vi "final.vi"() -> ()   [LabVIEW 2019]
uses:
  <vilib>/userdefined/High Color/IMAQdx.ctl
  <vilib>/DAQmx/write.llb/DAQmx Write (Digital 1D Bool NChan 1Samp 1Line).vi
  <vilib>/DAQmx/read.llb/DAQmx Read (Digital 1D Bool NChan 1Samp 1Line).vi
  <vilib>/Instr/_visa.llb/VISA Configure Serial Port (Instr).vi
  <vilib>/Utility/file.llb/Read Delimited Spreadsheet (DBL).vi
  <vilib>/DAQmx/miscellaneous.llb/DAQmx Fill In Error Info.vi
  <vilib>/Utility/file.llb/Write Delimited Spreadsheet (string).vi
  <vilib>/vision/driver/NI_Vision_Acquisition_Software.lvlib
  <vilib>/vision/NI_Vision_Development_Module.lvlib
panel:
  out "ready?":bool
  out "No Good Shot":bool
  in  "Mode":bool
  in  "Manual":u16(ring) items=["Straight", "Left", "Right", "Set Servo Angle"]
  in  "choose position":u8(slide) scale=0.0..255.0
  out "Servo":u8
  out "Image Out":T1(plugin-control)
  in  "shoot":bool
  in  "stop":bool
  # "Calculate"
  # "Set Manually"
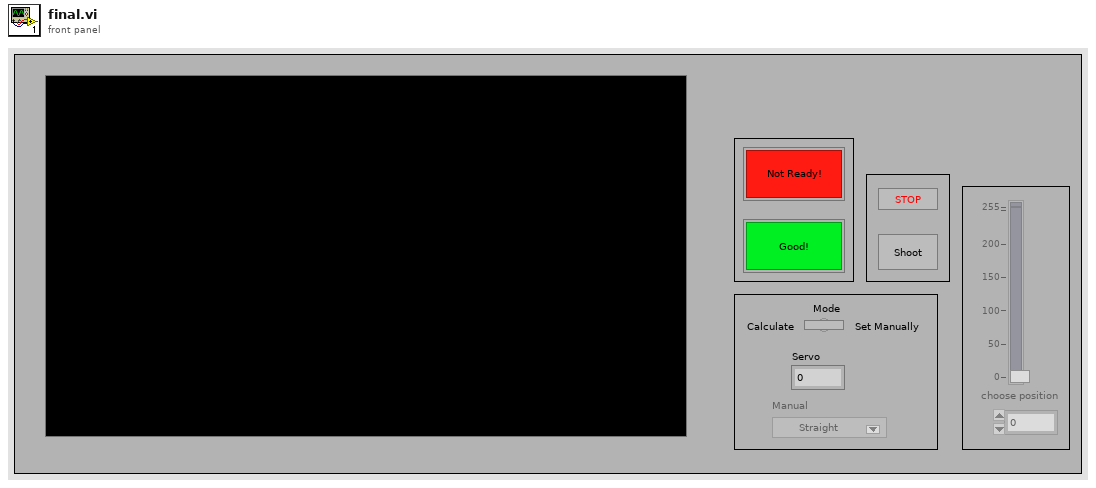
[diagram p1: front panel]
types:
  T1 = typedef "IMAQ Image.ctl" = refnum<image>
  T2 = typedef "IMAQdx.ctl" = refnum<k21>
  T3 = enum8{"Enabled", "Disabled", "Disabled and Grayed Out"}
  T4 = typedef "Image Type" = u32
  T5 = cluster{"Position":cluster{"x":sgl, "y":sgl}, "Angle":sgl, "Scale":sgl, "Score":sgl, "Bounding Box":cluster{"x":sgl, "y":sgl}[]}[]
  T6 = cluster{"Matches[0]":cluster{"Position":cluster{"x":sgl, "y":sgl}, "Angle":sgl, "Scale":sgl, "Score":sgl, "Bounding Box":cluster{"x":sgl, "y":sgl}[]}, "Matches[1]":cluster{"Position":cluster{"x":sgl, "y":sgl}, "Angle":sgl, "Scale":sgl, "Score":sgl, "Bounding Box":cluster{"x":sgl, "y":sgl}[]}, "Matches[2]":cluster{"Position":cluster{"x":sgl, "y":sgl}, "Angle":sgl, "Scale":sgl, "Score":sgl, "Bounding Box":cluster{"x":sgl, "y":sgl}[]}, "Matches[3]":cluster{"Position":cluster{"x":sgl, "y":sgl}, "Angle":sgl, "Scale":sgl, "Score":sgl, "Bounding Box":cluster{"x":sgl, "y":sgl}[]}, "Matches[4]":cluster{"Position":cluster{"x":sgl, "y":sgl}, "Angle":sgl, "Scale":sgl, "Score":sgl, "Bounding Box":cluster{"x":sgl, "y":sgl}[]}, "Matches[5]":cluster{"Position":cluster{"x":sgl, "y":sgl}, "Angle":sgl, "Scale":sgl, "Score":sgl, "Bounding Box":cluster{"x":sgl, "y":sgl}[]}, "Matches[6]":cluster{"Position":cluster{"x":sgl, "y":sgl}, "Angle":sgl, "Scale":sgl, "Score":sgl, "Bounding Box":cluster{"x":sgl, "y":sgl}[]}, "Matches[7]":cluster{"Position":cluster{"x":sgl, "y":sgl}, "Angle":sgl, "Scale":sgl, "Score":sgl, "Bounding Box":cluster{"x":sgl, "y":sgl}[]}, "Matches[8]":cluster{"Position":cluster{"x":sgl, "y":sgl}, "Angle":sgl, "Scale":sgl, "Score":sgl, "Bounding Box":cluster{"x":sgl, "y":sgl}[]}}
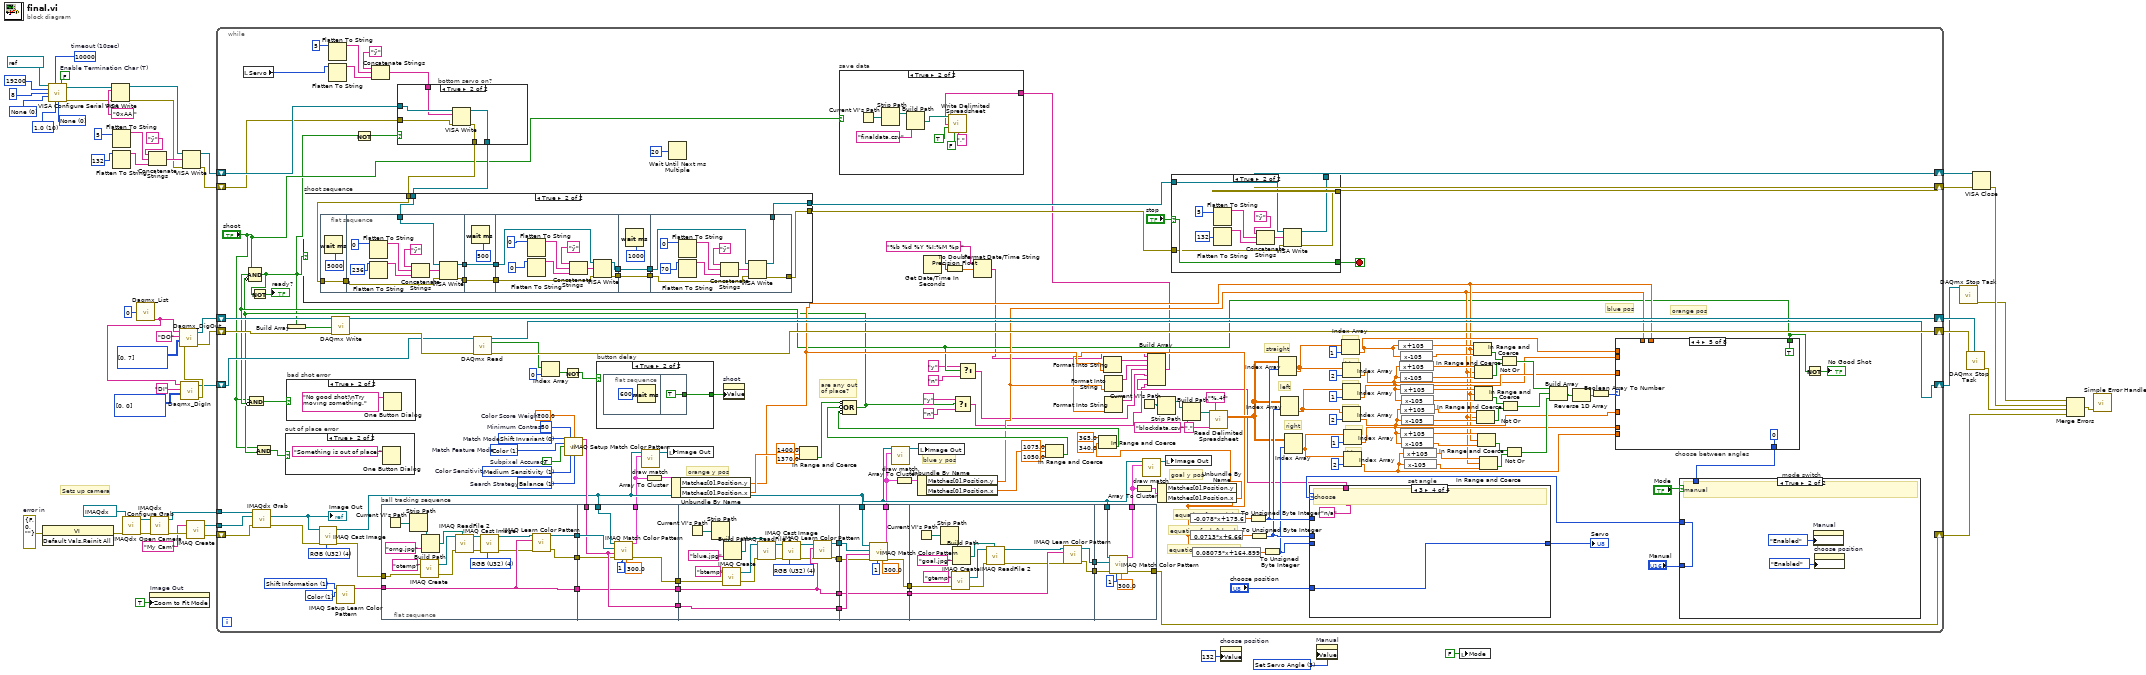
[diagram p0: block diagram]
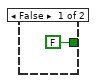
[diagram p2: hidden frame]
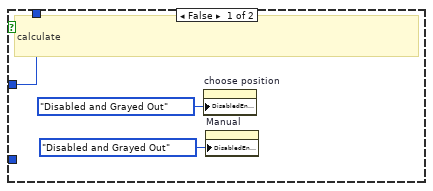
[diagram p6: hidden frame]
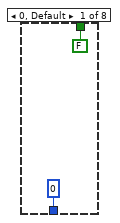
[diagram p7: hidden frame]
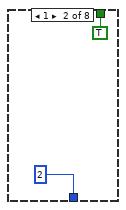
[diagram p8: hidden frame]
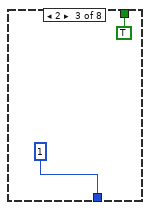
[diagram p9: hidden frame]
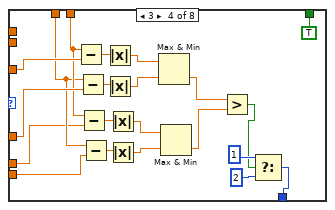
[diagram p10: hidden frame]
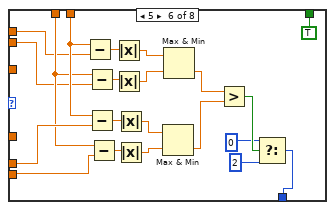
[diagram p11: hidden frame]
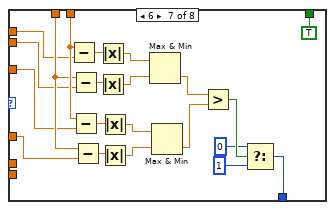
[diagram p12: hidden frame]
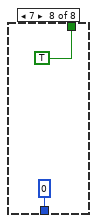
[diagram p13: hidden frame]
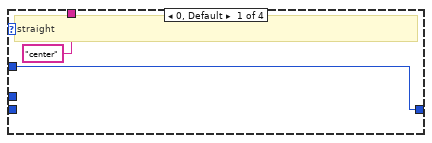
[diagram p14: hidden frame]
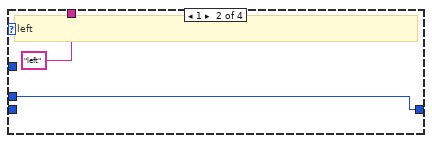
[diagram p15: hidden frame]
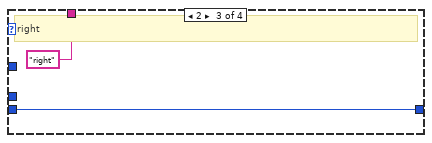
[diagram p16: hidden frame]
diagram:
  w9 = u16 3 items=["Straight", "Left", "Right", "Set Servo Angle"] ("select path")
  w38 = errorcluster {"status"=FALSE, "code"=0, "source"=""}  # error in
  w47 = u16 0 items=["None"=0, "XON/XOFF"=1, "RTS/CTS"=2, "DTR/DSR"=4] ("flow control")
  w48 = u16 10 items=["1.0"=10, "1.5"=15, "2.0"=20] ("stop bits")
  w49 = u16 0 items=["None", "Odd", "Even", "Mark", "Space"] ("parity")
  w53 = FALSE  # Enable Termination Char (T)
  w54 = u32 10000  # timeout (10sec)
  # "Sets up camera"
  n1 = invoke class="VI" method="Default Vals.Reinit All"(error in=w38) -> (error out=w37:errorcluster)  [unwired: 2 in, 2 out]
  n2 = call-poly "VISA Configure Serial Port"("VISA resource name"=refnum<visa-resource-name> "COM4", "timeout (10sec)"=w54, "Enable Termination\nChar (T)"=w53, "baud rate (9600)"=u32 19200 ("baud rate"), "data bits (8)"=u16 8 ("data bits"), "parity (0:none)"=w49, "stop bits (10: 1 bit)"=w48, "flow control (0:none)"=w47) -> ("VISA resource name out"=w45:refnum<visa-resource-name>, "error out"=w46:errorcluster)  [unwired: 1 in, 5 out]
  n3 = VISA Write(VISA resource name=w45, write buffer="0xAA ", error in (no error)=w46) -> (VISA resource name out=w15:refnum<visa-resource-name>, error out=w12:errorcluster)  [unwired: 1 out]
  n4 = Flatten To String(anything=u8 5) -> (data string=w19:string)  [unwired: 1 in, 4 out]
  n5 = Flatten To String(anything=u8 132) -> (data string=w21:string)  [unwired: 2 in, 3 out]
  n6 = call <vilib>:"IMAQdx Open Camera.vi"("error in"=w37, "Session In"=T2 "cam1") -> ("error out"=w35:errorcluster, "Session Out"=w36:T2)  [unwired: 8 in]
  n7 = call "Daqmx_List.vi"("Device Number n"=u8 0) -> ("NI-DAQmx Device Name n"=w5:tag)  [unwired: 3 out]
  n8 = Concatenate Strings("ÿ", w19, w21) -> (w20:string)
  n9 = property on="Image Out" class="ImageControl"("Zoom to Fit Mode"=TRUE) -> ()  [unwired: 2 in, 2 out]
  n10 = call <vilib>:"IMAQdx Configure Grab.vi"("error in"=w35, "Session In"=w36) -> ("error out"=w34:errorcluster, "Session Out"=w33:T2)  [unwired: 8 in]
  n11 = call "Daqmx_DigIn.vi"("Array of Ports, Lines"=i32[][] [[0, 0]] ("Outputs: Port, Line"), "Base Task Name"="DI", "DAQmx device name"=w5) -> ("error out"=w4:errorcluster, "Input Task Name"=w3:refnum<k21>)  [unwired: 2 in]
  n12 = call "Daqmx_DigOut.vi"("error in"=w4, "Array of Ports, Lines"=i32[][] [[0, 7]] ("Outputs: Port, Line"), "Base Task Name"="DO", "DAQmx device name"=w5) -> ("error out"=w27:errorcluster, "Output Task Name"=w39:refnum<k21>)  [unwired: 1 in]
  n13 = VISA Write(VISA resource name=w15, write buffer=w20, error in (no error)=w12) -> (VISA resource name out=w13:refnum<visa-resource-name>, error out=w14:errorcluster)  [unwired: 1 out]
  n14 = call "IMAQ Create"("Image Name"="My Cam", "error in (no error)"=w34) -> ("New Image"=w31:T1, "error out"=w29:errorcluster)  [unwired: 3 in]
  n15 = while {
    shift-right: [w162] -> w44
    shift-left: w13 -> [w221]
    shift-right: [w163] -> w43
    shift-left: w14 -> [w220]
    tunnel: w33 -> [w213]
    tunnel: w31 -> [w209]
    shift-right: [w170] -> w11
    shift-left: w29 -> [w210]
    shift-right: [w99] -> w26
    shift-left: w27 -> [w169]
    shift-right: [w168] -> w25
    shift-left: w39 -> [w215]
    shift-right: [w95] -> w2
    shift-left: w3 -> [w98]
    stop <- w166 stop-if-true
    w195 = u32 1 items=["Color and Shape", "Color", "Shape "] ("Feature Mode")
    w194 = u32 1 items=["All", "Shift Information", "Rotation Information"] ("Learn Mode")
    w201 = TRUE  # Subpixel Accuracy
    w202 = u32 1 items=["Color and Shape", "Color", "Shape"]  # Match Feature Mode
    w199 = u32 1 items=["Conservative", "Balance", "Aggressive", "Very Aggressive"]  # Search Strategy
    w204 = 50  # Minimum Contrast
    w203 = sgl 700.0  # Color Score Weight
    w200 = u32 1 items=["Low Sensitivity", "Medium Sensitivity", "High Sensitivity"]  # Color Sensitivity
    w205 = u32 0 items=["Shift Invariant", "Rotation Invariant"]  # Match Mode
    w211 = T4 4 items=["Grayscale (U8)", "Grayscale (I16)", "Grayscale (SGL)", "Complex (CSG)", "RGB (U32)", "HSL (U32)", "RGB (U64)", "Grayscale (U16)"] ("Image Type")
    # "are any out\nof place?"
    # "blue pos"
    # "orange pos"
    # "right"
    # "left"
    # "straight"
    # "blue"
    # "blue"
    # "orng"
    # "orng"
    # "blue"
    # "orng"
    # "equation for right bank"
    # "equation for left bank"
    # "equation for straight"
    # "goal y pos"
    # "blue y pos"
    # "orange y pos"
    n16 = local read "Servo"() -> (w160:u8)
    n17 = call <vilib>:"IMAQdx Grab.vi"("error in"=w210, "Image In"=w209, "Session In"=w213) -> ("error out"=w212:errorcluster, "Image Out"=w208:T1)  [unwired: 5 in, 2 out]
    "Image Out" <- w208
    n18 = call "IMAQ Cast Image"("Image Type"=w211, "error in (no error)"=w212, "Image Src"=w208) -> ("error out"=w176:errorcluster, "Image Dst Out"=w186:T1)  [unwired: 7 in]
    n19 = Flatten To String(anything=u8 5) -> (data string=w224:string)  [unwired: 1 in, 4 out]
    n20 = Flatten To String(anything=w160) -> (data string=w223:string)  [unwired: 1 in, 4 out]
    n21 = call "IMAQ Setup Learn Color Pattern"("Feature Mode"=w195, "Learn Mode"=w194) -> ("Learn Color Pattern Setup Data"=w193:string)  [unwired: 8 in, 1 out]
    n22 = Concatenate Strings("ÿ", w224, w223) -> (w219:string)
    n23 = flat-sequence "ball tracking sequence" {
      tunnel: [w347] -> w207
      tunnel: w193 -> [w346]
      tunnel: [w346] -> w191
      tunnel: w176 -> [w345]
      tunnel: [w341] -> w175
      tunnel: w186 -> [w364]
      tunnel: w207 -> [w365]
      tunnel: w198 -> [w362]
      tunnel: [w363] -> w182
      tunnel: [w362] -> w197
      tunnel: [w361] -> w192
      tunnel: w191 -> [w361]
      tunnel: w175 -> [w358]
      tunnel: [w357] -> w174
      tunnel: [w373] -> w206
      tunnel: w197 -> [w372]
      tunnel: [w372] -> w196
      tunnel: w192 -> [w371]
      tunnel: [w371] -> w189
      tunnel: w174 -> [w370]
      tunnel: [w366] -> w173
      tunnel: w186 -> [w390]
      tunnel: w206 -> [w391]
      tunnel: [w389] -> w180
      tunnel: w196 -> [w388]
      tunnel: [w385] -> w190
      tunnel: w189 -> [w385]
      tunnel: w173 -> [w384]
      tunnel: [w383] -> w172
      tunnel: w190 -> [w398]
      tunnel: [w397] -> w188
      tunnel: w172 -> [w395]
      tunnel: [w392] -> w171
      tunnel: [w409] -> w178
      tunnel: w186 -> [w408]
      tunnel: w188 -> [w407]
      tunnel: w171 -> [w406]
      tunnel: [w405] -> w170
      frame #0 {
        w352 = T4 4 items=["Grayscale (U8)", "Grayscale (I16)", "Grayscale (SGL)", "Complex (CSG)", "RGB (U32)", "HSL (U32)", "RGB (U64)", "Grayscale (U16)"] ("Image Type")
        n24 = Current VI's Path() -> (path=w351:path)
        n25 = Strip Path(path=w351) -> (stripped path=w350:path)  [unwired: 1 out]
        n26 = call "IMAQ Create"("Image Name"="otemp", "error in (no error)"=w345) -> ("New Image"=w353:T1, "error out"=w344:errorcluster)  [unwired: 3 in]
        n27 = Build Path(base path=w350, name or relative path="orng.jpg") -> (appended path=w355:path)
        n28 = call "IMAQ ReadFile 2"("File Path"=w355, "error in (no error)"=w344, "Image"=w353) -> ("error out"=w343:errorcluster, "Image Out"=w348:T1)  [unwired: 4 in, 3 out]
        n29 = call "IMAQ Cast Image"("Image Type"=w352, "error in (no error)"=w343, "Image Src"=w348) -> ("error out"=w342:errorcluster, "Image Dst Out"=w349:T1)  [unwired: 7 in]
        n30 = call "IMAQ Learn Color Pattern"("error in (no error)"=w342, "Learn Color Pattern Setup Data"=w346, "Image"=w349) -> ("error out"=w341:errorcluster, "Template Image Out"=w347:T1)  [unwired: 7 in]
      }
      frame #1 {
        n31 = call "IMAQ Match Color Pattern"("Minimum Match Score"=sgl 300.0, "Number of Matches Requested"=1, "error in (no error)"=w358, "Match Color Pattern Setup Data"=w362, "Template Image"=w365, "Image"=w364) -> ("error out"=w357:errorcluster, "Matches"=w363:T5)  [unwired: 3 in, 1 out]
      }
      frame #2 {
        w378 = T4 4 items=["Grayscale (U8)", "Grayscale (I16)", "Grayscale (SGL)", "Complex (CSG)", "RGB (U32)", "HSL (U32)", "RGB (U64)", "Grayscale (U16)"] ("Image Type")
        n32 = Current VI's Path() -> (path=w377:path)
        n33 = Strip Path(path=w377) -> (stripped path=w376:path)  [unwired: 1 out]
        n34 = call "IMAQ Create"("Image Name"="btemp", "error in (no error)"=w370) -> ("New Image"=w379:T1, "error out"=w369:errorcluster)  [unwired: 3 in]
        n35 = Build Path(base path=w376, name or relative path="blue.jpg") -> (appended path=w381:path)
        n36 = call "IMAQ ReadFile 2"("File Path"=w381, "error in (no error)"=w369, "Image"=w379) -> ("error out"=w368:errorcluster, "Image Out"=w375:T1)  [unwired: 4 in, 3 out]
        n37 = call "IMAQ Cast Image"("Image Type"=w378, "error in (no error)"=w368, "Image Src"=w375) -> ("error out"=w367:errorcluster, "Image Dst Out"=w374:T1)  [unwired: 7 in]
        n38 = call "IMAQ Learn Color Pattern"("error in (no error)"=w367, "Learn Color Pattern Setup Data"=w371, "Image"=w374) -> ("error out"=w366:errorcluster, "Template Image Out"=w373:T1)  [unwired: 7 in]
      }
      frame #3 {
        n39 = call "IMAQ Match Color Pattern"("Minimum Match Score"=sgl 300.0, "Number of Matches Requested"=1, "error in (no error)"=w384, "Match Color Pattern Setup Data"=w388, "Template Image"=w391, "Image"=w390) -> ("error out"=w383:errorcluster, "Matches"=w389:T5)  [unwired: 3 in, 1 out]
      }
      frame #4 {
        n40 = Current VI's Path() -> (path=w400:path)
        n41 = Strip Path(path=w400) -> (stripped path=w399:path)  [unwired: 1 out]
        n42 = call "IMAQ Create"("Image Name"="gtemp", "error in (no error)"=w395) -> ("New Image"=w401:T1, "error out"=w394:errorcluster)  [unwired: 3 in]
        n43 = Build Path(base path=w399, name or relative path="goal.jpg") -> (appended path=w403:path)
        n44 = call "IMAQ ReadFile 2"("File Path"=w403, "error in (no error)"=w394, "Image"=w401) -> ("error out"=w393:errorcluster, "Image Out"=w396:T1)  [unwired: 4 in, 3 out]
        n45 = call "IMAQ Learn Color Pattern"("error in (no error)"=w393, "Learn Color Pattern Setup Data"=w398, "Image"=w396) -> ("error out"=w392:errorcluster, "Template Image Out"=w397:T1)  [unwired: 7 in]
      }
      frame #5 {
        n46 = call "IMAQ Match Color Pattern"("Minimum Match Score"=sgl 300.0, "Number of Matches Requested"=1, "error in (no error)"=w406, "Template Image"=w407, "Image"=w408) -> ("error out"=w405:errorcluster, "Matches"=w409:T5)  [unwired: 4 in, 1 out]
      }
    }
    n47 = call "IMAQ Setup Match Color Pattern"("Match Mode"=w205, "Minimum Contrast"=w204, "Color Score Weight"=w203, "Match Feature Mode"=w202, "Subpixel Accuracy"=w201, "Color Sensitivity"=w200, "Search Strategy"=w199) -> ("Match Color Pattern Setup Data"=w198:string)  [unwired: 7 in, 1 out]
    n48 = call "draw match.vi"("Matches"=w182, "Image"=w186) -> ("Image Out"=w184:T1)  [unwired: 9 in]
    n49 = Array To Cluster(array=w182) -> (cluster=w181:T6)
    n50 = local write "Image Out"(w184) -> ()
    n51 = Wait Until Next ms Multiple(millisecond multiple=u32 20 ("millisecond timer value")) -> ()  [unwired: 1 out]
    n52 = Unbundle By Name(w181) -> ("Matches[0].Position.y"=w80:sgl, "Matches[0].Position.x"=w93:sgl)
    n53 = In Range and Coerce(upper limit=sgl 1400.0, x=w93, lower limit=sgl 1370.0) -> (In Range?=w84:bool)  [unwired: 1 out]
    n54 = call "draw match.vi"("Matches"=w180, "Image"=w186) -> ("Image Out"=w183:T1)  [unwired: 9 in]
    n55 = Array To Cluster(array=w180) -> (cluster=w179:T6)
    n56 = Unbundle By Name(w179) -> ("Matches[0].Position.y"=w79:sgl, "Matches[0].Position.x"=w90:sgl)
    n57 = local write "Image Out"(w183) -> ()
    n58 = Get Date/Time In Seconds() -> (seconds since 1Jan1904=w61:timestamp)
    n59 = To Double Precision Float(number=w61) -> (double precision float=w60:dbl)
    n60 = Format Date/Time String(time format string (%c)="%b %d %Y %I:%M %p ", seconds (now)=w60) -> (date/time string=w62:string)  [unwired: 1 in]
    n61 = In Range and Coerce(upper limit=sgl 1075.0, x=w90, lower limit=sgl 1050.0) -> (In Range?=w83:bool)  [unwired: 1 out]
    n62 = Format Into String(w80) -> (resulting string=w77:string)  [unwired: 3 in, 1 out]
    n63 = Format Into String(w79) -> (resulting string=w76:string)  [unwired: 3 in, 1 out]
    n64 = Array To Cluster(array=w178) -> (cluster=w177:T6)
    n65 = Current VI's Path() -> (path=w155:path)
    n66 = call "draw match.vi"("Matches"=w178, "Image"=w186) -> ("Image Out"=w185:T1)  [unwired: 9 in]
    n67 = Unbundle By Name(w177) -> ("Matches[0].Position.y"=w78:sgl, "Matches[0].Position.x"=w87:sgl)
    n68 = In Range and Coerce(upper limit=sgl 365.0, x=w87, lower limit=sgl 340.0) -> (In Range?=w82:bool)  [unwired: 1 out]
    n69 = Compound Arithmetic op=OR(invert w84, invert w83, invert w82) -> (w67:bool)
    n70 = And(x="shoot", y=w67) -> (x .and. y?=w81:bool)
    n71 = case "out of place error" shown="True" w81 {
      frame False {
      }
      frame True {
        n72 = One Button Dialog(message="Something is out of place.") -> ()  [unwired: 1 in, 1 out]
      }
    }
    n73 = Select(t="y", s=w67, f="n") -> (s? t:f=w66:string)
    n74 = Format Into String(w78) -> (resulting string=w75:string)  [unwired: 3 in, 1 out]
    n75 = Strip Path(path=w155) -> (stripped path=w154:path)  [unwired: 1 out]
    n76 = local write "Image Out"(w185) -> ()
    n77 = Build Path(base path=w154, name or relative path="blockdata.csv") -> (appended path=w152:path)
    n78 = expression code="-0.078*x+175.6"(w78) -> (w161:sgl)
    n79 = expression code="0.0713*x+6.66"(w78) -> (w159:sgl)
    n80 = expression code="0.08075*x+164.899"(w78) -> (w158:sgl)
    n81 = call-poly <vilib>:"Read Delimited Spreadsheet.vi"("file path (dialog if empty)"=w152, "format (%.3f)"="%.4f", "delimiter (\\t)"="," ("delimiter (\\t)")) -> ("all rows"=w147:dbl[][])  [unwired: 7 in, 5 out]
    n82 = To Unsigned Byte Integer(number=w161) -> (unsigned 8bit integer=w149:u8)
    n83 = To Unsigned Byte Integer(number=w159) -> (unsigned 8bit integer=w148:u8)
    n84 = To Unsigned Byte Integer(number=w158) -> (unsigned 8bit integer=w146:u8)
    n85 = Index Array(array=w147, index (row)=w149) -> (element=w144:dbl[])  [unwired: 1 in]
    n86 = Index Array(array=w147, index (row)=w148) -> (element=w136:dbl[])  [unwired: 1 in]
    n87 = Index Array(array=w147, index (row)=w146) -> (element=w135:dbl[])  [unwired: 1 in]
    n88 = Index Array(array=w144, index=1) -> (element=w120:dbl)
    n89 = Index Array(array=w144, index=2) -> (element=w103:dbl)
    n90 = Index Array(array=w136, index=1) -> (element=w104:dbl)
    n91 = Index Array(array=w136, index=2) -> (element=w105:dbl)
    n92 = Index Array(array=w135, index=1) -> (element=w106:dbl)
    n93 = Index Array(array=w135, index=2) -> (element=w107:dbl)
    n94 = expression code="x+105"(w120) -> (w119:dbl)
    n95 = expression code="x+105"(w103) -> (w117:dbl)
    n96 = expression code="x-105"(w120) -> (w118:dbl)
    n97 = expression code="x+105"(w104) -> (w115:dbl)
    n98 = expression code="x+105"(w106) -> (w111:dbl)
    n99 = expression code="x-105"(w103) -> (w116:dbl)
    n100 = expression code="x+105"(w105) -> (w113:dbl)
    n101 = expression code="x-105"(w104) -> (w114:dbl)
    n102 = expression code="x-105"(w105) -> (w112:dbl)
    n103 = expression code="x-105"(w106) -> (w110:dbl)
    n104 = expression code="x+105"(w107) -> (w109:dbl)
    n105 = expression code="x-105"(w107) -> (w108:dbl)
    n106 = In Range and Coerce(upper limit=w119, x=w80, lower limit=w118) -> (In Range?=w142:bool)  [unwired: 1 out]
    n107 = In Range and Coerce(upper limit=w115, x=w80, lower limit=w114) -> (In Range?=w140:bool)  [unwired: 1 out]
    n108 = In Range and Coerce(upper limit=w117, x=w79, lower limit=w116) -> (In Range?=w141:bool)  [unwired: 1 out]
    n109 = In Range and Coerce(upper limit=w113, x=w79, lower limit=w112) -> (In Range?=w139:bool)  [unwired: 1 out]
    n110 = In Range and Coerce(upper limit=w111, x=w80, lower limit=w110) -> (In Range?=w138:bool)  [unwired: 1 out]
    n111 = In Range and Coerce(upper limit=w109, x=w79, lower limit=w108) -> (In Range?=w137:bool)  [unwired: 1 out]
    n112 = Not Or(1:w141, 2:w142) -> (0:w125:bool)
    n113 = Not Or(1:w139, 2:w140) -> (0:w124:bool)
    n114 = Not Or(1:w137, 2:w138) -> (0:w123:bool)
    n115 = Build Array(w125, w124, w123) -> (w122:bool[])
    n116 = Reverse 1D Array(array=w122) -> (reversed array=w121:bool[])
    n117 = Boolean Array To Number(Boolean array=w121) -> (number=w130:u32)
    n118 = case "choose between angles" shown="4" w130 {
      tunnel: [0 ("f") 2 1 w272 0 w282 w303 0 ("f")] -> w126
      tunnel: w79 -> [_ _ _ w262 _ w288 w308 _]
      tunnel: w80 -> [_ _ _ w263 _ w289 w309 _]
      tunnel: w120 -> [_ _ _ _ _ w287 w307 _]
      tunnel: w103 -> [_ _ _ _ _ w286 w306 _]
      tunnel: w104 -> [_ _ _ w269 _ _ w305 _]
      tunnel: w105 -> [_ _ _ w268 _ _ w304 _]
      tunnel: w106 -> [_ _ _ w261 _ w291 _ _]
      tunnel: w107 -> [_ _ _ w260 _ w290 _ _]
      tunnel: [FALSE TRUE TRUE TRUE TRUE TRUE TRUE TRUE] -> w74
      frame 0, Default {
      }
      frame 1 {
      }
      frame 2 {
      }
      frame 3 {
        n119 = Subtract(x=w263, y=w269) -> (x-y=w267:dbl)
        n120 = Subtract(x=w262, y=w268) -> (x-y=w266:dbl)
        n121 = Subtract(x=w263, y=w261) -> (x-y=w265:dbl)
        n122 = Subtract(x=w262, y=w260) -> (x-y=w264:dbl)
        n123 = Absolute Value(x=w267) -> (abs(x)=w258:dbl)
        n124 = Absolute Value(x=w266) -> (abs(x)=w257:dbl)
        n125 = Absolute Value(x=w265) -> (abs(x)=w255:dbl)
        n126 = Absolute Value(x=w264) -> (abs(x)=w254:dbl)
        n127 = Max & Min(x=w258, y=w257) -> (min(x,y)=w256:dbl)  [unwired: 1 out]
        n128 = Max & Min(x=w255, y=w254) -> (min(x,y)=w253:dbl)  [unwired: 1 out]
        n129 = Greater?(x=w256, y=w253) -> (0:w259:bool)
        n130 = Select(t=1, s=w259, f=2) -> (s? t:f=w272:i32)
      }
      frame 4 {
      }
      frame 5 {
        n131 = Subtract(x=w289, y=w287) -> (x-y=w292:dbl)
        n132 = Subtract(x=w288, y=w286) -> (x-y=w293:dbl)
        n133 = Subtract(x=w289, y=w291) -> (x-y=w294:dbl)
        n134 = Subtract(x=w288, y=w290) -> (x-y=w295:dbl)
        n135 = Absolute Value(x=w292) -> (abs(x)=w278:dbl)
        n136 = Absolute Value(x=w293) -> (abs(x)=w279:dbl)
        n137 = Absolute Value(x=w294) -> (abs(x)=w281:dbl)
        n138 = Absolute Value(x=w295) -> (abs(x)=w280:dbl)
        n139 = Max & Min(x=w281, y=w280) -> (min(x,y)=w276:dbl)  [unwired: 1 out]
        n140 = Max & Min(x=w278, y=w279) -> (min(x,y)=w277:dbl)  [unwired: 1 out]
        n141 = Greater?(x=w277, y=w276) -> (0:w285:bool)
        n142 = Select(t=0, s=w285, f=2) -> (s? t:f=w282:i32)
      }
      frame 6 {
        n143 = Subtract(x=w309, y=w307) -> (x-y=w313:dbl)
        n144 = Subtract(x=w308, y=w306) -> (x-y=w314:dbl)
        n145 = Subtract(x=w309, y=w305) -> (x-y=w315:dbl)
        n146 = Subtract(x=w308, y=w304) -> (x-y=w316:dbl)
        n147 = Absolute Value(x=w313) -> (abs(x)=w299:dbl)
        n148 = Absolute Value(x=w314) -> (abs(x)=w300:dbl)
        n149 = Absolute Value(x=w315) -> (abs(x)=w302:dbl)
        n150 = Absolute Value(x=w316) -> (abs(x)=w301:dbl)
        n151 = Max & Min(x=w299, y=w300) -> (min(x,y)=w298:dbl)  [unwired: 1 out]
        n152 = Max & Min(x=w302, y=w301) -> (min(x,y)=w297:dbl)  [unwired: 1 out]
        n153 = Greater?(x=w298, y=w297) -> (0:w312:bool)
        n154 = Select(t=0, s=w312, f=1) -> (s? t:f=w303:i32)
      }
      frame 7 {
      }
    }
    n155 = Compound Arithmetic op=AND("shoot", w74, invert w67) -> (w58:bool)
    n156 = Compound Arithmetic op=AND("shoot", invert w74) -> (w102:bool)
    n157 = Not(x=w58) -> (.not. x?=→"ready?":bool)
    n158 = case "bad shot error" shown="True" w102 {
      frame False {
      }
      frame True {
        n159 = One Button Dialog(message="No good shot!\nTry moving something.") -> ()  [unwired: 1 in, 1 out]
      }
    }
    n160 = Build Array(w58) -> (w214:bool[])
    n161 = call-poly <vilib>:"DAQmx Write.vi"("task/channels in"=w215, "data"=w214, "error in"=w169) -> ("task out"=w168:refnum<k21>, "error out"=w100:errorcluster)  [unwired: 10 in, 1 out]
    n162 = Not(x=w58) -> (.not. x?=w216:bool)
    n163 = case "bottom servo on?" shown="True" w216 {
      tunnel: w221 -> [w412 w418]
      tunnel: w220 -> [w413 w417]
      tunnel: w219 -> [_ w416]
      tunnel: [w413 w415] -> w218
      tunnel: [w412 w414] -> w217
      frame False {
      }
      frame True {
        n164 = VISA Write(VISA resource name=w418, write buffer=w416, error in (no error)=w417) -> (VISA resource name out=w414:refnum<visa-resource-name>, error out=w415:errorcluster)  [unwired: 1 out]
      }
    }
    n165 = case "shoot sequence" shown="True" w58 {
      tunnel: w217 -> [w420 w433]
      tunnel: w218 -> [w419 w429]
      tunnel: [w420 w422] -> w165
      tunnel: [w419 w421] -> w164
      frame False {
      }
      frame True {
        n166 = flat-sequence {
          tunnel: w429 -> [w435]
          tunnel: [w435] -> w423
          tunnel: w433 -> [w440]
          tunnel: [w438] -> w432
          tunnel: [w436] -> w427
          tunnel: w423 -> [w437]
          tunnel: w432 -> [w447]
          tunnel: [w447] -> w431
          tunnel: [w446] -> w428
          tunnel: w427 -> [w446]
          tunnel: w431 -> [w452]
          tunnel: [w451] -> w430
          tunnel: w428 -> [w450]
          tunnel: [w449] -> w426
          tunnel: w430 -> [w459]
          tunnel: w426 -> [w460]
          tunnel: [w460] -> w425
          tunnel: [w459] -> w424
          tunnel: w425 -> [w465]
          tunnel: w424 -> [w464]
          tunnel: [w463] -> w422
          tunnel: [w462] -> w421
          frame #0 {
            n167 = Wait (ms)(milliseconds to wait=u32 5000) -> ()  [unwired: 1 out]
          }
          frame #1 {
            n168 = Flatten To String(anything=u8 0) -> (data string=w444:string)  [unwired: 1 in, 4 out]
            n169 = Flatten To String(anything=u8 236) -> (data string=w443:string)  [unwired: 2 in, 3 out]
            n170 = Concatenate Strings("ÿ", w444, w443) -> (w439:string)
            n171 = VISA Write(VISA resource name=w440, write buffer=w439, error in (no error)=w437) -> (VISA resource name out=w438:refnum<visa-resource-name>, error out=w436:errorcluster)  [unwired: 1 out]
          }
          frame #2 {
            n172 = Wait (ms)(milliseconds to wait=u32 500) -> ()  [unwired: 1 out]
          }
          frame #3 {
            n173 = Flatten To String(anything=u8 0) -> (data string=w457:string)  [unwired: 1 in, 4 out]
            n174 = Flatten To String(anything=u8 0) -> (data string=w456:string)  [unwired: 2 in, 3 out]
            n175 = Concatenate Strings("ÿ", w457, w456) -> (w453:string)
            n176 = VISA Write(VISA resource name=w452, write buffer=w453, error in (no error)=w450) -> (VISA resource name out=w451:refnum<visa-resource-name>, error out=w449:errorcluster)  [unwired: 1 out]
          }
          frame #4 {
            n177 = Wait (ms)(milliseconds to wait=u32 1000) -> ()  [unwired: 1 out]
          }
          frame #5 {
            n178 = Flatten To String(anything=u8 0) -> (data string=w470:string)  [unwired: 1 in, 4 out]
            n179 = Flatten To String(anything=u8 70) -> (data string=w469:string)  [unwired: 2 in, 3 out]
            n180 = Concatenate Strings("ÿ", w470, w469) -> (w466:string)
            n181 = VISA Write(VISA resource name=w464, write buffer=w466, error in (no error)=w465) -> (VISA resource name out=w463:refnum<visa-resource-name>, error out=w462:errorcluster)  [unwired: 1 out]
          }
        }
      }
    }
    n182 = call-poly <vilib>:"DAQmx Read.vi"("task/channels in"=w98, "error in"=w100) -> ("task out"=w95:refnum<k21>, "data"=w96:bool[], "error out"=w99:errorcluster)  [unwired: 11 in]
    n183 = Index Array(array=w96, index=0) -> (element=w94:bool)
    n184 = Not(x=w94) -> (.not. x?=w57:bool)
    n185 = case "button delay" shown="True" w57 {
      tunnel: [FALSE w227] -> w56
      frame False {
      }
      frame True {
        n186 = flat-sequence {
          tunnel: [TRUE] -> w227
          frame #0 {
            n187 = Wait (ms)(milliseconds to wait=u32 600) -> ()  [unwired: 1 out]
          }
          frame #1 {
          }
        }
      }
    }
    n188 = property on="shoot" class="Bool (strict)"("Value"=w56) -> ()  [unwired: 2 in, 2 out]
    n189 = Select(t="y", s=w74, f="n") -> (s? t:f=w71:string)
    n190 = case shown="True" "stop" {
      selector: "stop" -> [w329 w334]
      tunnel: [w329 w334] -> w166
      tunnel: w165 -> [w327 w333]
      tunnel: w164 -> [w328 w332]
      tunnel: [w328 w331] -> w163
      tunnel: [w327 w330] -> w162
      frame False {
      }
      frame True {
        n191 = Flatten To String(anything=u8 5) -> (data string=w338:string)  [unwired: 1 in, 4 out]
        n192 = Flatten To String(anything=u8 132) -> (data string=w340:string)  [unwired: 2 in, 3 out]
        n193 = Concatenate Strings("ÿ", w338, w340) -> (w339:string)
        n194 = VISA Write(VISA resource name=w333, write buffer=w339, error in (no error)=w332) -> (VISA resource name out=w330:refnum<visa-resource-name>, error out=w331:errorcluster)  [unwired: 1 out]
      }
    }
    n195 = case "mode switch" shown="True" "Mode" {
      tunnel: "Manual" -> [_ w245]
      tunnel: [w242 w245] -> w127
      tunnel: w126 -> [w242 _]
      frame False {
        # "calculate"
        n196 = property on="choose position" class="Slide (strict)"("DisabledEnum"=T3."Disabled and Grayed Out" ("Disabled")) -> ()  [unwired: 2 in, 2 out]
        n197 = property on="Manual" class="Ring (strict)"("DisabledEnum"=T3."Disabled and Grayed Out" ("Disabled")) -> ()  [unwired: 2 in, 2 out]
      }
      frame True {
        # "manual"
        n198 = property on="Manual" class="Ring (strict)"("DisabledEnum"=T3."Enabled" ("Disabled")) -> ()  [unwired: 2 in, 2 out]
        n199 = property on="choose position" class="Slide (strict)"("DisabledEnum"=T3."Enabled" ("Disabled")) -> ()  [unwired: 2 in, 2 out]
      }
    }
    n200 = case "set angle" shown="3" w127 {
      tunnel: "choose position" -> [_ _ _ w326]
      tunnel: [w320 w322 w324 w326] -> w156
      tunnel: w146 -> [_ _ w324 _]
      tunnel: w148 -> [_ w322 _ _]
      tunnel: w149 -> [w320 _ _ _]
      tunnel: ["center" "left" "right" "n/a"] -> w70
      frame 0, Default {
        # "straight"
      }
      frame 1 {
        # "left"
      }
      frame 2 {
        # "right"
      }
      frame 3 {
        # "choose"
      }
    }
    "Servo" <- w156
    n201 = Build Array(w62, w77, w76, w75, w71, w70, w66) -> (w65:string[])
    n202 = case "save data" shown="True" "shoot" {
      tunnel: w65 -> [_ w230]
      frame False {
      }
      frame True {
        n203 = Current VI's Path() -> (path=w237:path)
        n204 = Strip Path(path=w237) -> (stripped path=w236:path)  [unwired: 1 out]
        n205 = Build Path(base path=w236, name or relative path="finaldata.csv") -> (appended path=w234:path)
        n206 = call-poly <vilib>:"Write Delimited Spreadsheet.vi"("file path (dialog if empty)"=w234, "1D data"=w230, "append to file? (new file:F)"=TRUE, "transpose? (no:F)"=FALSE, "delimiter (\\t)"="," ("delimiter (\\t)")) -> ()  [unwired: 9 in, 2 out]
      }
    }
    n207 = Not(x=w74) -> (.not. x?=→"No Good Shot":bool)
  }
  n208 = property on="choose position" class="Slide (strict)"("Value"=u8 132 ("choose position")) -> ()  [unwired: 2 in, 2 out]
  n209 = property on="Manual" class="Ring (strict)"("Value"=w9) -> ()  [unwired: 2 in, 2 out]
  n210 = local write "Mode"(FALSE ("Mode")) -> ()
  n211 = call <vilib>:"DAQmx Stop Task.vi"("task/channels in"=w2) -> ("error out"=w1:errorcluster)  [unwired: 13 in, 1 out]
  n212 = call <vilib>:"DAQmx Stop Task.vi"("task/channels in"=w25, "error in"=w26) -> ("error out"=w23:errorcluster)  [unwired: 12 in, 1 out]
  n213 = VISA Close(VISA resource name=w44, error in (no error)=w43) -> (error out=w22:errorcluster)
  n214 = Merge Errors(w1, w22, w23, w11) -> (w24:errorcluster)
  n215 = call <vilib>:"Simple Error Handler.vi"("error in (no error)"=w24) -> ()  [unwired: 4 in, 5 out]
